vi "Shuffle.vi"() -> ()   [LabVIEW 2013]
panel:
  out "Array 2":cluster{string, "Joint Values":dbl[]}[][](array[cluster])
  in  "Array":cluster{string, "Joint Values":dbl[]}[][](array[cluster])
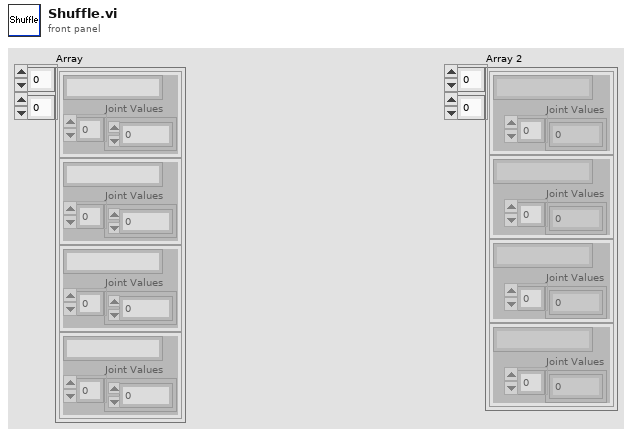
[diagram p1: front panel]
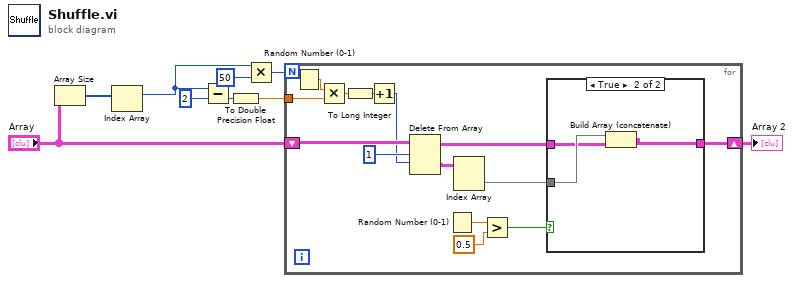
[diagram p0: block diagram]
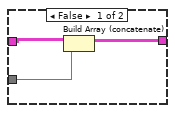
[diagram p2: hidden frame]
diagram:
  n1 = Array Size(array="Array") -> (size(s)=w5:i32[])
  n2 = Index Array(array=w5) -> (element=w1:i32)  [unwired: 1 in]
  n3 = Subtract(x=w1, y=2) -> (x-y=w3:i32)
  n4 = To Double Precision Float(number=w3) -> (double precision float=w7:dbl)
  n5 = Multiply(x=w1, y=50) -> (x*y=w8:i32)
  n6 = for {
    N: w8 -> [_]
    tunnel: w7 -> [w22]
    shift-right: [w11] -> w4
    shift-left: "Array" -> [w20]
    n7 = Random Number (0-1)() -> (number: 0 to 1=w23:dbl)
    n8 = Multiply(x=w23, y=w22) -> (x*y=w21:dbl)
    n9 = To Long Integer(number=w21) -> (32bit integer=w17:i32)
    n10 = Increment(x=w17) -> (x+1=w10:i32)
    n11 = Delete From Array(array=w20, length=1, index (row)=w10) -> (deleted portion=w18:cluster{string, "Joint Values":dbl[]}[][], array with subset deleted=w13:cluster{string, "Joint Values":dbl[]}[][])  [unwired: 1 in]
    n12 = Random Number (0-1)() -> (number: 0 to 1=w16:dbl)
    n13 = Index Array(array=w18) -> (element=w12:cluster{string, "Joint Values":dbl[]}[])  [unwired: 2 in]
    n14 = Greater?(x=w16, y=0.5) -> (0:w14:bool)
    n15 = case shown="True" w14 {
      tunnel: w13 -> [w25 w27]
      tunnel: w12 -> [w26 w29]
      tunnel: [w24 w28] -> w11
      frame False {
        n16 = Build Array (concatenate)(w25, w26) -> (w24:cluster{string, "Joint Values":dbl[]}[][])
      }
      frame True {
        n17 = Build Array (concatenate)(w29, w27) -> (w28:cluster{string, "Joint Values":dbl[]}[][])
      }
    }
  }
  "Array 2" <- w4
